vi "Sgraph-Close.vi"(8 "error in (no error)":errorcluster) -> (0 "error out":errorcluster)   [LabVIEW 2020, in "Gserver.lvclass"]
doc: "Close the Sgraph service"
uses:
  Gserver.lvclass
  controls/Typedef_Gviewer-Query.ctl
  controls/Typedef_QueryType.ctl
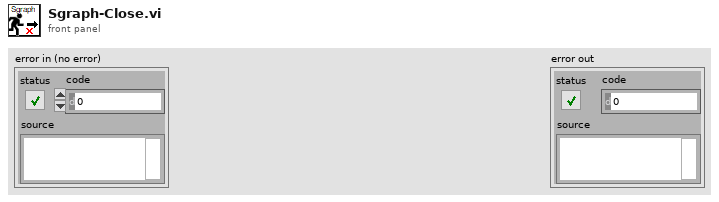
[diagram p1: front panel]
types:
  T1 = typedef "Gserver.lvclass/Typedef_QueryType.ctl" = enum16{"Subscribe", "DataRequest", "RequestAllTags", "RequestIniPath", "FAMMstarted", "SetClientOptions", "GviewerUpdate", "OpenNewGraph", "CloseClient", "CloseAllClients", "Close Gserver", "OpenMemoryMap", "MeMapDataRequest", "MeMapDataResponse"}
  T2 = typedef "Gserver.lvclass/Typedef_Gviewer-Query.ctl" = cluster{"Query_type":T1, "data":variant, "Source":string, "Time Stamp":timestamp}
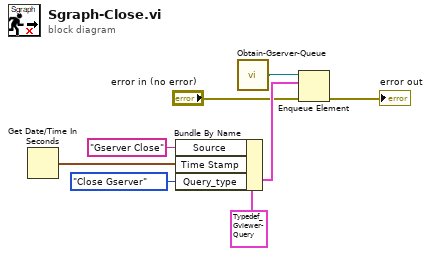
[diagram p0: block diagram]
diagram:
  n1 = Get Date/Time In Seconds() -> (seconds since 1Jan1904=w4:timestamp)
  n2 = Bundle By Name(cluster=T2 {"Query_type"=enum."Subscribe", "data"=variant, "Source"="", "Time Stamp"=timestamp(0 s since 1904-01-01)} ("element"), "Source"="Gserver Close", "Time Stamp"=w4, "Query_type"=Typedef_QueryType."Close Gserver") -> (w6:T2)
  n3 = call "Obtain-Gserver-Queue.vi"() -> ("Gserver Queue"=w8:refnum<queue>)  [unwired: 7 in]
  n4 = Enqueue Element(queue=w8, element=w6, error in (no error)="error in (no error)") -> (error out=→"error out":errorcluster)  [unwired: 1 in, 2 out]
